vi "str2Date.vi"(11 "String":string="27-MAR-19") -> (3 "Time Stamp":timestamp)   [LabVIEW 2018, in "Controller.lvlib"]
uses:
  Controller.lvlib
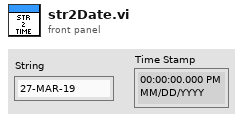
[diagram p1: front panel]
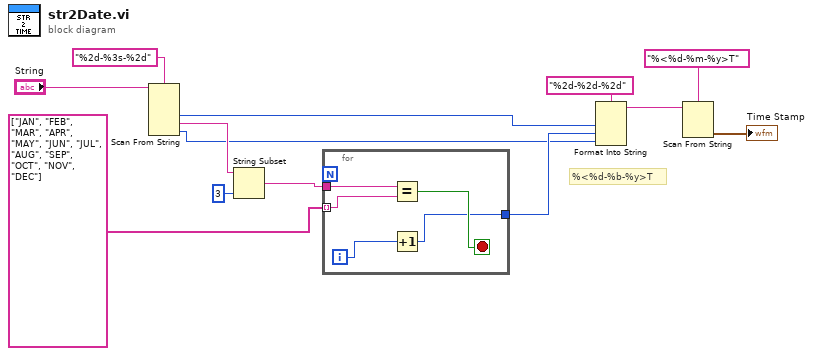
[diagram p0: block diagram]
diagram:
  # "%<%d-%b-%y>T"
  n1 = Scan From String(format string="%2d-%3s-%2d", input string="String") -> (output 1=w3:i32, output 2=w8:string, output 3=w1:i32)  [unwired: 5 in, 3 out]
  n2 = String Subset(string=w8, length (rest)=3 ("length (rest)")) -> (substring=w6:string)  [unwired: 1 in]
  n3 = for {
    tunnel: string[] ["JAN", "FEB", "MAR", "APR", "MAY", "JUN", "JUL", "AUG", "SEP", "OCT", "NOV", "DEC"] -> [w16] mode=indexing
    tunnel: w6 -> [w18]
    tunnel: [w14] -> w2
    i -> [w15]
    stop <- w17 stop-if-true
    n4 = Equal?(x=w18, y=w16) -> (x = y?=w17:bool)
    n5 = Increment(x=w15) -> (x+1=w14:i32)
  }
  n6 = Format Into String(format string="%2d-%2d-%2d", w3, w2, w1) -> (resulting string=w4:string)  [unwired: 2 in, 1 out]
  n7 = Scan From String(format string="%<%d-%m-%y>T", input string=w4) -> (output 1=→"Time Stamp":timestamp)  [unwired: 3 in, 3 out]
